vi "Stop.vi"(8 "error in (no error)":errorcluster, 11 "bt_System in":refnum<class "bt_System.lvclass">) -> (0 "error out":errorcluster, 3 "bt_System out":refnum<class "bt_System.lvclass">)   [LabVIEW 2021, in "BT.lvlib" / "bt_System.lvclass"]
uses:
  bt_System.lvclass
  bt_System.lvclass/bt_System.ctl
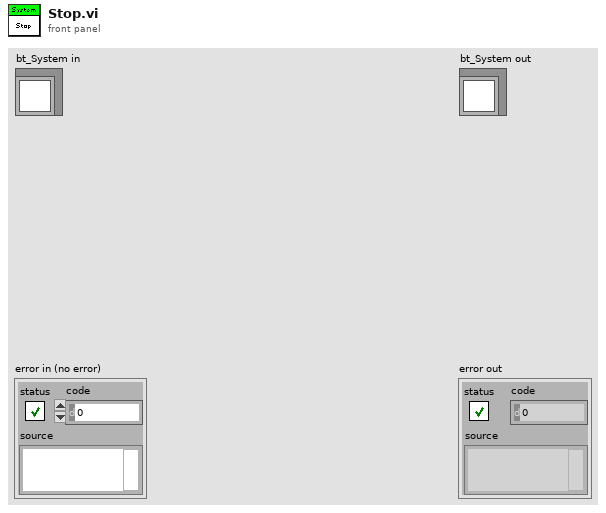
[diagram p1: front panel]
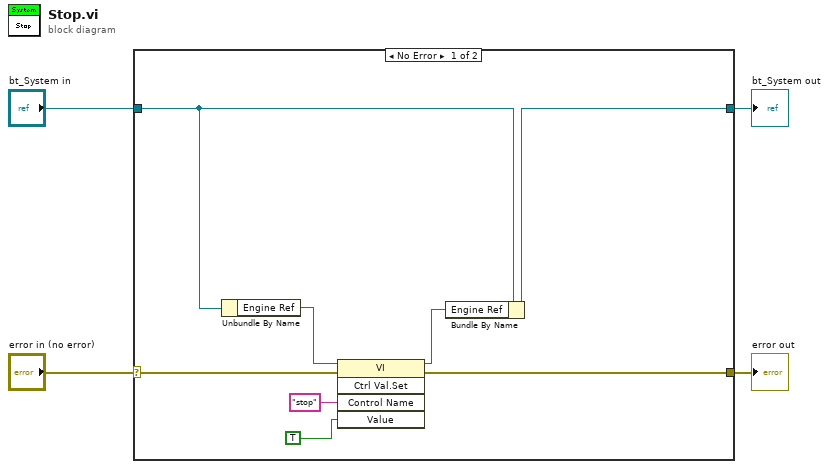
[diagram p0: block diagram]
diagram:
  n1 = case shown="No Error" "error in (no error)" {
    selector: "error in (no error)" -> [w11 w14]
    tunnel: [w7 w14] -> w3
    tunnel: [w6 w13] -> w1
    tunnel: "bt_System in" -> [w12 w13]
    frame No Error {
      n2 = Unbundle By Name(w12) -> ("Engine Ref"=w10:refnum<vi>)
      n3 = invoke class="VI" method="Ctrl Val.Set"(reference=w10, error in=w11, "Control Name"="stop", "Value"=TRUE) -> (reference out=w5:refnum<vi>, error out=w7:errorcluster)  [unwired: 1 in, 3 out]
      n4 = Bundle By Name(cluster=w12, "Engine Ref"=w5) -> (w6:refnum<class "bt_System.lvclass">)
    }
    frame Error {
    }
  }
  "error out" <- w3
  "bt_System out" <- w1
